vi "addOrReplaceLabviewConditionalSymbol.vi"() -> ()   [LabVIEW 2023]
uses:
  <userlib>/_OpenG.lib/array/array.llb/Slice 1D Array (String)__ogtk.vi
  <vilib>/Wiresmith Technology/G CLI/CLI Class/CLI.lvclass
panel:
  out "String":string
  out "map":map{string, string}(c390)
  in  "error in":errorcluster
  # "Locals"
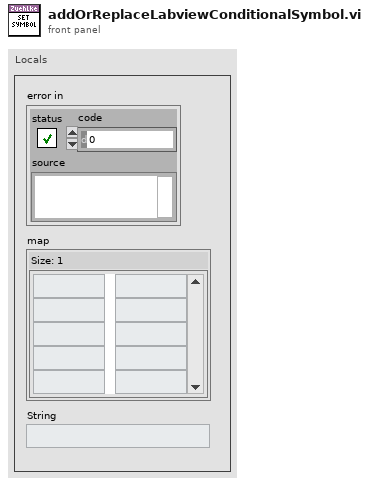
[diagram p1: front panel]
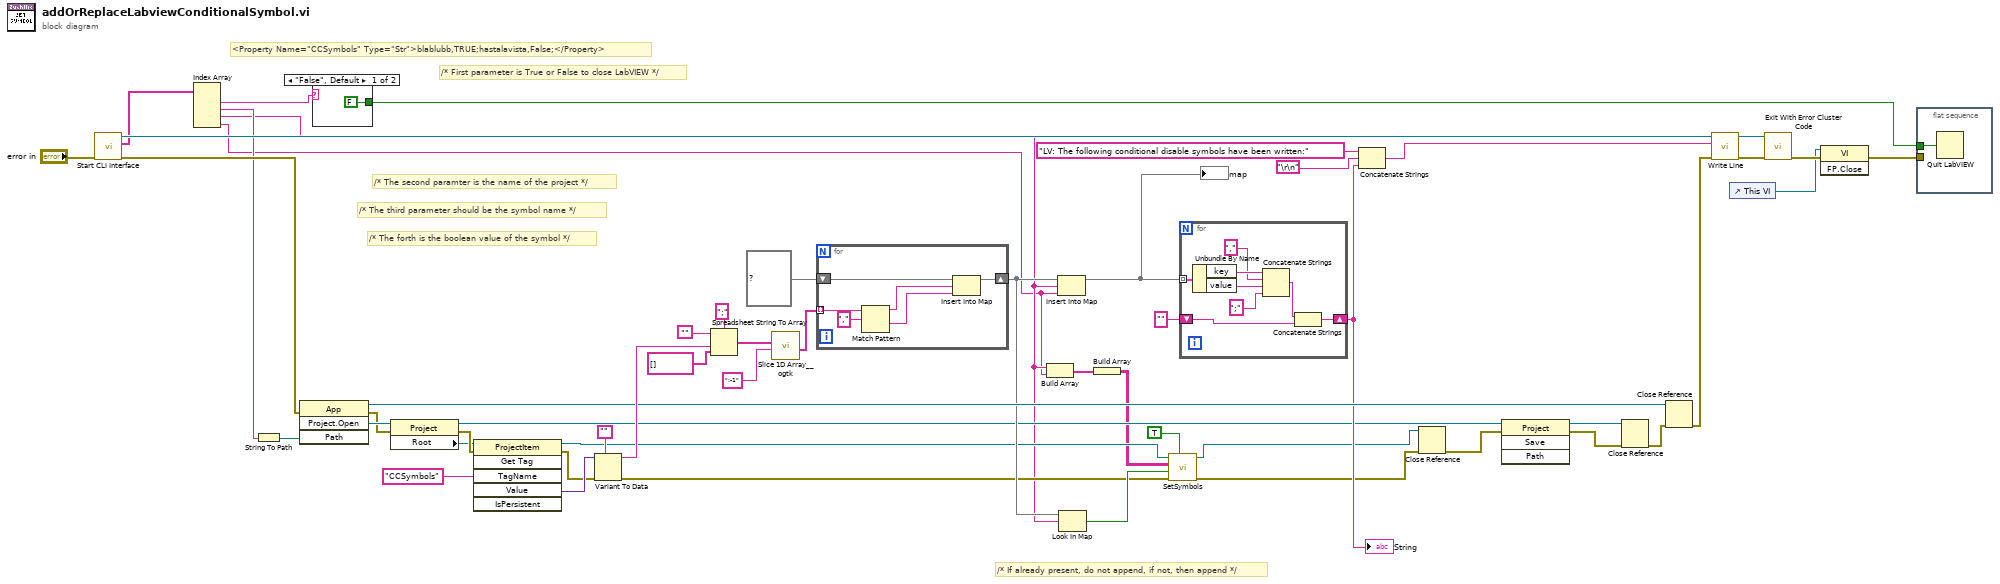
[diagram p0: block diagram]
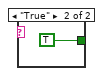
[diagram p2: hidden frame]
diagram:
  # "/* If already present, do not append, if not, then append */"
  # "/* The second paramter is the name of the project */"
  # "/* The forth is the boolean value of the symbol */"
  # "/* The third parameter should be the symbol name */"
  # "/* First parameter is True or False to close LabVIEW */"
  # "<Property Name=\"CCSymbols\" Type=\"Str\">blablubb,TRUE;hastalavista,False;</Property>"
  n1 = call <vilib>:"Start CLI Interface.vi"("error in (no error)"="error in") -> ("error out"=w17:errorcluster, "Custom Parameters"=w23:string[], "CLI out"=w28:refnum<class "CLI.lvclass">)  [unwired: 7 in, 1 out]
  n2 = Index Array(array=w23) -> (element #1=w30:string, element #2=w13:string, element #3=w3:string, element #4=w2:string)  [unwired: 4 in]
  n3 = String To Path(string=w13) -> (path=w14:path)
  n4 = invoke class="App" method="Project.Open"(error in=w17, "Path"=w14) -> (reference out=w36:refnum<vi>, error out=w51:errorcluster, "Project:Open"=w52:refnum<vi>)  [unwired: 2 in, 1 out]
  n5 = case shown="\"False\", Default" w30 {
    tunnel: [FALSE TRUE] -> w29
    frame "False", Default {
    }
    frame "True" {
    }
  }
  n6 = property class="Project"(reference=w52, error in=w51) -> (reference out=w8:refnum<vi>, error out=w50:errorcluster, "Root"=w44:refnum<vi>)
  n7 = invoke class="ProjectItem" method="Get Tag"(reference=w44, error in=w50, "TagName"="CCSymbols" ("Tag Name")) -> (reference out=w7:refnum<vi>, error out=w38:errorcluster, "Value"=w53:variant)  [unwired: 3 in, 3 out]
  n8 = Variant To Data(error in=w38, type="", Variant=w53) -> (data=w49:string, error out=w10:errorcluster)
  n9 = Spreadsheet String To Array(delimiter (Tab)=";", format string="", spreadsheet string=w49, array type (2D Dbl)=string[] []) -> (array=w33:string[])
  n10 = call-poly <userlib>:"Slice 1D Array__ogtk.vi"("slice"=":-1", "array"=w33) -> ("subarray (array[i:j])"=w31:string[])  [unwired: 5 in]
  n11 = for {
    tunnel: w31 -> [w60] mode=indexing
    shift-right: [w58] -> w12
    shift-left: map{string, string} {} ("map") -> [w59]
    n12 = Match Pattern(string=w60, regular expression=",") -> (before substring=w57:string, after substring=w56:string)  [unwired: 3 out]
    n13 = Insert Into Map(map in=w59, key=w57, value=w56) -> (map out=w58:map{string, string})  [unwired: 2 out]
  }
  n14 = Build Array(w3, w2) -> (w4:string[])
  n15 = Insert Into Map(map in=w12, key=w3, value=w2) -> (map out=w39:map{string, string})  [unwired: 2 out]
  "map" <- w39
  n16 = Look In Map(map=w12, key=w3) -> (key not found?=w11:bool)  [unwired: 1 in, 1 out]
  n17 = Build Array(w4) -> (w1:string[][])
  n18 = call <resource>:"SetSymbols.vi"("Is Persistant? (FALSE)"=TRUE, "error in"=w10, "Append? (TRUE)"=w11, "Symbol Value Pairs"=w1, "Project Item"=w7) -> ("error out"=w9:errorcluster, "Project Item"=w6:refnum<vi>)  [unwired: 5 in]
  n19 = for {
    tunnel: w39 -> [w69] mode=indexing
    shift-right: [w62] -> w18
    shift-left: "" -> [w63]
    n20 = Unbundle By Name(w69) -> ("key"=w68:string, "value"=w66:string)
    n21 = Concatenate Strings(w68, "," ("string"), w66, ";" ("string")) -> (w64:string)
    n22 = Concatenate Strings(w64, w63) -> (w62:string)
  }
  "String" <- w18
  n23 = Concatenate Strings("LV: The following conditional disable symbols have been written:" ("string"), "\r\n", w18) -> (w19:string)
  n24 = Close Reference(reference=w6, error in (no error)=w9) -> (error out=w37:errorcluster)
  n25 = invoke class="Project" method="Save"(reference=w8, error in=w37) -> (reference out=w42:refnum<vi>, error out=w41:errorcluster)  [unwired: 2 in, 2 out]
  n26 = Close Reference(reference=w42, error in (no error)=w41) -> (error out=w35:errorcluster)
  n27 = Close Reference(reference=w36, error in (no error)=w35) -> (error out=w15:errorcluster)
  n28 = call <vilib>:"Write Line.vi"("error in (no error)"=w15, "Text to Write"=w19, "CLI in"=w28) -> ("error out"=w22:errorcluster, "CLI out"=w27:refnum<class "CLI.lvclass">)  [unwired: 7 in]
  n29 = control-ref of="This VI"() -> (w16:refnum<vi>)
  n30 = call <vilib>:"Exit With Error Cluster Code.vi"("error in (no error)"=w22, "CLI in"=w27) -> ("error out"=w21:errorcluster)  [unwired: 9 in]
  n31 = invoke class="VI" method="FP.Close"(reference=w16, error in=w21) -> (error out=w20:errorcluster)  [unwired: 1 in, 2 out]
  n32 = flat-sequence {
    tunnel: w29 -> [w70]
    tunnel: w20 -> [_]
    frame #0 {
      n33 = Quit LabVIEW(quit? (T)=w70) -> ()
    }
  }
